vi "initial_collection.vi"(1 "Input":dbl, 2 "Flag":bool) -> (0 "Ouput":dbl)   [LabVIEW 2021]
uses:
  <vilib>/ptbypt/NI_PtbyPt.lvlib
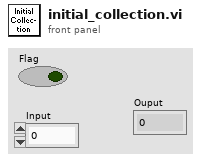
[diagram p1: front panel]
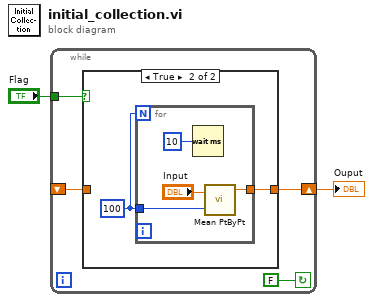
[diagram p0: block diagram]
diagram:
  n1 = while {
    tunnel: "Flag" -> [w6]
    shift-right: [w4] -> w1
    shift-left: _ -> [w3]
    stop <- FALSE continue-if-true
    n2 = case shown="True" w6 {
      tunnel: [w7 w8] -> w4
      tunnel: w3 -> [w7 _]
      frame False {
      }
      frame True {
        w9 = 100
        n3 = for {
          N: w9 -> [_]
          tunnel: w9 -> [w11]
          tunnel: [w10] -> w8
          n4 = Wait (ms)(milliseconds to wait=u32 10) -> ()  [unwired: 1 out]
          n5 = call <vilib>:"Mean PtByPt.vi"("x"="Input", "sample length"=w11) -> ("mean"=w10:dbl)  [unwired: 2 in, 1 out]
        }
      }
    }
  }
  "Ouput" <- w1
